vi "test_communicator_main.vi"(8 "error in (no error)":errorcluster) -> (0 "error out":errorcluster)   [LabVIEW 2020, in "horiba.test.lvlib"]
uses:
  horiba.test.lvlib
  424cda72-e919-4ae5-9e87-5671caa6f1b6.vi
  Classes/Communicator/Communicator.lvclass
  90e1af07-9827-437a-8956-efd347084262.vi
panel:
  # "Connector Pane"
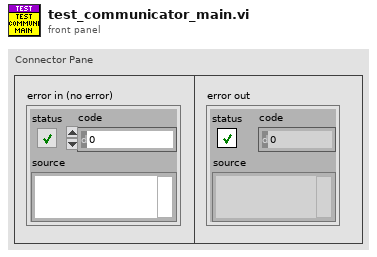
[diagram p1: front panel]
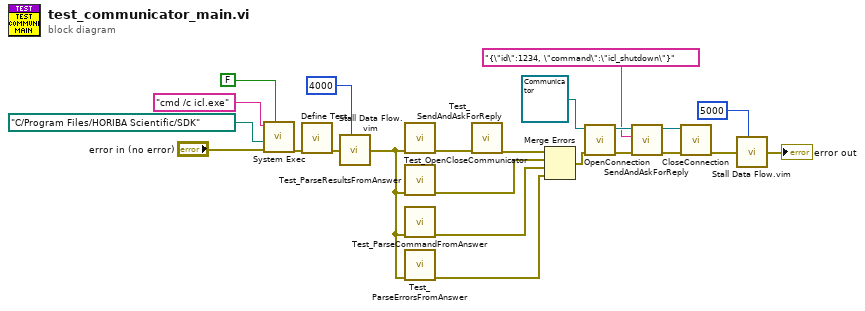
[diagram p0: block diagram]
diagram:
  n1 = call <vilib>:"System Exec.vi"("wait until completion? (T)"=FALSE, "error in (no error)"="error in (no error)", "working directory"=path "C:/Program Files/HORIBA Scientific/SDK", "command line"="cmd /c icl.exe") -> ("error out"=w20:errorcluster)  [unwired: 4 in, 3 out]
  n2 = call <vilib>:"Define Test.vi"("error in (no error)"=w20) -> ("error out"=w18:errorcluster)  [unwired: 9 in, 1 out]
  n3 = call "Stall Data Flow.vim"("value in"=w18, "milliseconds to wait"=u32 4000) -> ("value out"=w16:errorcluster)  [unwired: 1 out]
  n4 = call "Test_OpenCloseCommunicator.vi"("error in (no error)"=w16) -> ("error out"=w17:errorcluster)  [unwired: 10 in]
  n5 = call "Test_ParseResultsFromAnswer.vi"("error in (no error)"=w16) -> ("error out"=w8:errorcluster)  [unwired: 10 in]
  n6 = call "Test_ParseCommandFromAnswer.vi"("error in (no error)"=w16) -> ("error out"=w7:errorcluster)  [unwired: 10 in]
  n7 = call "Test_ParseErrorsFromAnswer.vi"("error in (no error)"=w16) -> ("error out"=w6:errorcluster)  [unwired: 10 in]
  n8 = call "Test_SendAndAskForReply.vi"("error in (no error)"=w17) -> ("error out"=w9:errorcluster)  [unwired: 10 in]
  n9 = Merge Errors(w9, w8, w7, w6) -> (w10:errorcluster)
  n10 = call-dynamic "OpenConnection.vi"("error in (no error)"=w10, "Communicator in"=refnum<class "Communicator.lvclass"> refnum) -> ("error out"=w14:errorcluster, "Communicator out"=w15:refnum<class "Communicator.lvclass">)  [unwired: 7 in, 1 out]
  n11 = call-dynamic "SendAndAskForReply.vi"("error in (no error)"=w14, "String to be sent"="{\"id\":1234, \"command\":\"icl_shutdown\"}", "Communicator in"=w15) -> ("error out"=w12:errorcluster, "Communicator out"=w13:refnum<class "Communicator.lvclass">)  [unwired: 6 in, 1 out]
  n12 = call-dynamic "CloseConnection.vi"("error in (no error)"=w12, "Communicator in"=w13) -> ("error out"=w5:errorcluster)  [unwired: 8 in, 1 out]
  n13 = call "Stall Data Flow.vim"("value in"=w5, "milliseconds to wait"=u32 5000) -> ("value out"=→"error out":errorcluster)  [unwired: 1 out]
